vi "X-Y Go(Global).vi"() -> ()   [LabVIEW 2010]
panel:
  out "y-axis":bool
  out "x-axis":bool
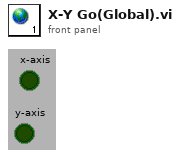
[diagram p1: front panel]
diagram:
